vi "ABAPI Dist Exclude Files From Linker Info.vi"(5 "LinkerInfo":T1(array[cluster]), 6 "top-level files":path[](array[path]), 7 "directories of excluded files":string[](array[string])) -> (1 "LinkerInfoOut":T1(array[cluster]), 3 "files excluded":bool)   [LabVIEW 2020]
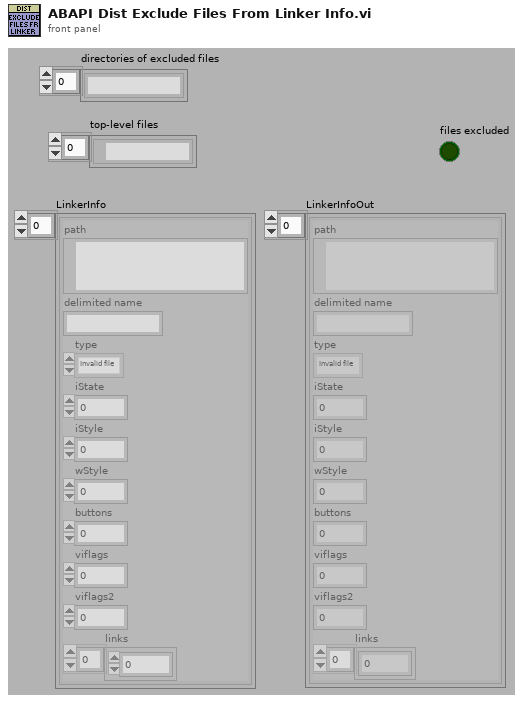
[diagram p1: front panel]
types:
  T1 = cluster{"path":path, "delimited name":string, "type":enum32{"Invalid file", "Unknown type", "Instrument", "Control", "Polymorphic VI", "Project", "Library", "LVClass", "XControl", "XNode", "Shared library", ".NET assembly", "ActiveX interface", "CIN", "Run-time menu", "Palette menu", "Help file", "LLB"}, "iState":u32, "iStyle":u16, "wStyle":u16, "buttons":u16, "viflags":u32, "viflags2":u32, "links":u32[]}[]
  T2 = cluster{"path":path, "delimited name":string, "type":enum32{"Invalid file", "Unknown type", "Instrument", "Control", "Polymorphic VI", "Project", "Library", "LVClass", "XControl", "XNode", "Shared library", ".NET assembly", "ActiveX interface", "CIN", "Run-time menu", "Palette menu", "Help file", "LLB"}, "iState":u32, "iStyle":u16, "wStyle":u16, "buttons":u16, "viflags":u32, "viflags2":u32, "links":u32[]}
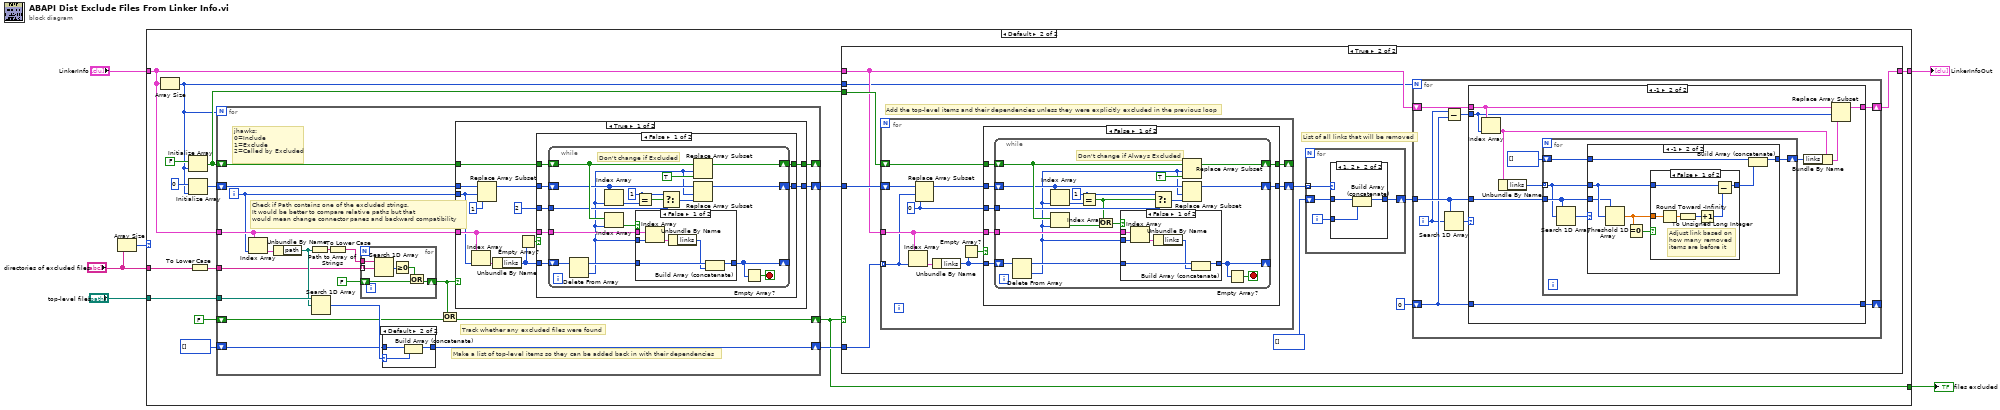
[diagram p0: block diagram]
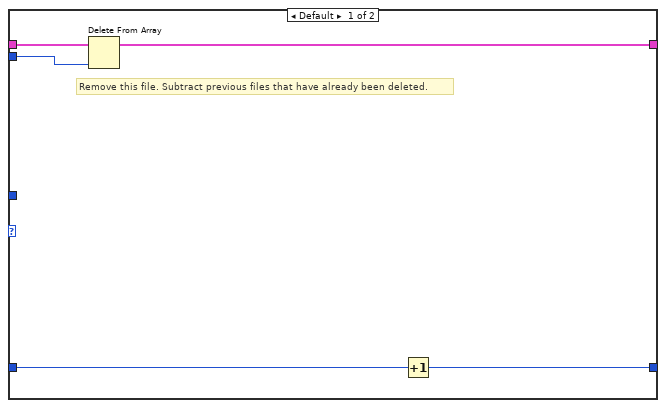
[diagram p4: hidden frame]
diagram:
  n1 = Array Size(array="directories of excluded files") -> (size(s)=w4:i32)
  n2 = case shown="Default" w4 {
    tunnel: "top-level files" -> [_ w19]
    tunnel: [w7 w14] -> w6
    tunnel: "LinkerInfo" -> [w7 w11]
    tunnel: [_ w9] -> w1
    tunnel: "directories of excluded files" -> [_ w8]
    frame 0 {
    }
    frame Default {
      n3 = Array Size(array=w11) -> (size(s)=w13:i32)
      n4 = Initialize Array(FALSE, w13) -> (w16:bool[])
      n5 = Initialize Array(0, w13) -> (w21:i32[])
      n6 = To Lower Case(string=w8) -> (all lower case string=w10:string[])
      n7 = for {
        N: w13 -> [_]
        shift-right: [w138] -> w17
        shift-left: w21 -> [w147]
        shift-right: [w139] -> _
        shift-left: w16 -> [w148]
        tunnel: w11 -> [w146]
        tunnel: w19 -> [w144]
        shift-right: [w142] -> w15
        shift-left: i32[] [] -> [w141]
        shift-right: [w136] -> w9
        shift-left: FALSE -> [w137]
        tunnel: w10 -> [w131]
        i -> [w140]
        # "jhawks:\n0=Include\n1=Exclude\n2=Called by Excluded"
        # "Make a list of top-level items so they can be added back in with their dependencies"
        # "Track whether any excluded files were found"
        # "Check if Path contains one of the excluded strings.\nIt would be better to compare relative paths but that\nwould mean change connector panes and backward compatibility"
        n8 = Index Array(array=w146, index=w140) -> (element=w145:T2)
        n9 = Unbundle By Name(w145) -> ("path"=w132:path)
        n10 = Path to Array of Strings(0:w132) -> (2:w133:string[])  [unwired: 1 out]
        n11 = Search 1D Array(1D array=w144, element=w132) -> (index of element=w143:i32)  [unwired: 1 in]
        n12 = To Lower Case(string=w133) -> (all lower case string=w130:string[])
        n13 = for {
          tunnel: w131 -> [w149] mode=indexing
          tunnel: w130 -> [w152]
          shift-right: [w154] -> w134
          shift-left: FALSE -> [w153]
          n14 = Search 1D Array(1D array=w152, element=w149) -> (index of element=w151:i32)  [unwired: 1 in]
          n15 = Greater Or Equal To 0?(x=w151) -> (x >= 0?=w150:bool)
          n16 = Or(x=w150, y=w153) -> (x .or. y?=w154:bool)
        }
        n17 = case shown="Default" w143 {
          selector: w143 -> [_ w158]
          tunnel: [w155 w157] -> w142
          tunnel: w141 -> [w155 w156]
          frame -1 {
          }
          frame Default {
            n18 = Build Array (concatenate)(w156, w158) -> (w157:i32[])
          }
        }
        n19 = Or(x=w134, y=w137) -> (x .or. y?=w136:bool)
        n20 = case shown="True" w134 {
          tunnel: w146 -> [w165 _]
          tunnel: w147 -> [w169 w205]
          tunnel: [w166 w205] -> w138
          tunnel: w148 -> [w164 w204]
          tunnel: [w163 w204] -> w139
          tunnel: w140 -> [w161 _]
          frame True {
            n21 = Index Array(array=w165, index=w161) -> (element=w170:T2)
            n22 = Replace Array Subset(array=w169, new element=1 ("new element/subarray"), index=w161) -> (w168:i32[])
            n23 = Unbundle By Name(w170) -> ("links"=w160:u32[])
            n24 = Empty Array?(array=w160) -> (empty?=w159:bool)
            n25 = case shown="False" w159 {
              tunnel: w160 -> [w177 _]
              tunnel: w168 -> [w176 w202]
              tunnel: [w175 w202] -> w166
              tunnel: w165 -> [w174 _]
              tunnel: w164 -> [w173 w203]
              tunnel: [w172 w203] -> w163
              tunnel: 2 ("new element/subarray") -> [w171 _]
              frame False {
                n26 = while {
                  shift-right: [w194] -> w175
                  shift-left: w176 -> [w184]
                  tunnel: w171 -> [w180]
                  shift-right: [w190] -> _
                  shift-left: w177 -> [w193]
                  tunnel: w174 -> [w192]
                  shift-right: [w188] -> w172
                  shift-left: w173 -> [w186]
                  stop <- w189 stop-if-true
                  w181 = 1 ("x")
                  # "Don't change if Excluded"
                  n27 = Delete From Array(array=w193) -> (deleted portion=w178:u32, array with subset deleted=w191:u32[])  [unwired: 2 in]
                  n28 = Index Array(array=w184, index=w178) -> (element=w183:i32)
                  n29 = Index Array(array=w186, index=w178) -> (element=w185:bool)
                  n30 = case shown="False" w185 {
                    tunnel: w192 -> [w200 _]
                    tunnel: w178 -> [w199 _]
                    tunnel: w191 -> [w197 w201]
                    tunnel: [w195 w201] -> w190
                    frame False {
                      n31 = Index Array(array=w200, index=w199) -> (element=w198:T2)
                      n32 = Unbundle By Name(w198) -> ("links"=w196:u32[])
                      n33 = Build Array (concatenate)(w197, w196) -> (w195:u32[])
                    }
                    frame True {
                    }
                  }
                  n34 = Equal?(x=w181, y=w183) -> (x = y?=w182:bool)
                  n35 = Select(t=w181, s=w182, f=w180) -> (s? t:f=w179:i32)
                  n36 = Replace Array Subset(array=w186, new element=TRUE ("new element/subarray"), index=w178) -> (w188:bool[])
                  n37 = Replace Array Subset(array=w184, new element=w179, index=w178) -> (w194:i32[])
                  n38 = Empty Array?(array=w190) -> (empty?=w189:bool)
                }
              }
              frame True {
              }
            }
          }
          frame False {
          }
        }
      }
      n39 = case shown="True" w9 {
        tunnel: w17 -> [_ w33]
        tunnel: w16 -> [_ w32]
        tunnel: w15 -> [_ w31]
        tunnel: w11 -> [w23 w27]
        tunnel: [w23 w26] -> w14
        tunnel: w13 -> [_ w25]
        frame False {
        }
        frame True {
          # "List of all links that will be removed"
          # "Add the top-level items and their dependencies unless they were explicitly excluded in the previous loop"
          n40 = for {
            tunnel: w27 -> [w94]
            shift-right: [w95] -> w30
            shift-left: w33 -> [w91]
            shift-right: [w88] -> _
            shift-left: w32 -> [w89]
            tunnel: w31 -> [w87] mode=indexing
            w92 = 0 ("new element/subarray")
            n41 = Index Array(array=w94, index=w87) -> (element=w93:T2)
            n42 = Replace Array Subset(array=w91, new element=w92, index=w87) -> (w90:i32[])
            n43 = Unbundle By Name(w93) -> ("links"=w86:u32[])
            n44 = Empty Array?(array=w86) -> (empty?=w85:bool)
            n45 = case shown="False" w85 {
              tunnel: [w102 w128] -> w95
              tunnel: w94 -> [w101 _]
              tunnel: w86 -> [w100 _]
              tunnel: w92 -> [w99 _]
              tunnel: w90 -> [w98 w128]
              tunnel: w89 -> [w97 w129]
              tunnel: [w96 w129] -> w88
              frame False {
                n46 = while {
                  shift-right: [w118] -> w102
                  shift-left: w98 -> [w109]
                  tunnel: w99 -> [w108]
                  shift-right: [w115] -> _
                  shift-left: w100 -> [w120]
                  tunnel: w101 -> [w117]
                  shift-right: [w114] -> w96
                  shift-left: w97 -> [w112]
                  stop <- w119 stop-if-true
                  w111 = 1 ("x")
                  # "Don't change if Always Excluded"
                  n47 = Delete From Array(array=w120) -> (deleted portion=w106:u32, array with subset deleted=w116:u32[])  [unwired: 2 in]
                  n48 = Index Array(array=w109, index=w106) -> (element=w110:i32)
                  n49 = Index Array(array=w112, index=w106) -> (element=w105:bool)
                  n50 = Equal?(x=w111, y=w110) -> (x = y?=w103:bool)
                  n51 = Or(x=w103, y=w105) -> (x .or. y?=w104:bool)
                  n52 = case shown="False" w104 {
                    tunnel: w117 -> [w126 _]
                    tunnel: w106 -> [w125 _]
                    tunnel: w116 -> [w123 w127]
                    tunnel: [w121 w127] -> w115
                    frame False {
                      n53 = Index Array(array=w126, index=w125) -> (element=w124:T2)
                      n54 = Unbundle By Name(w124) -> ("links"=w122:u32[])
                      n55 = Build Array (concatenate)(w123, w122) -> (w121:u32[])
                    }
                    frame True {
                    }
                  }
                  n56 = Select(t=w111, s=w103, f=w108) -> (s? t:f=w107:i32)
                  n57 = Replace Array Subset(array=w112, new element=TRUE ("new element/subarray"), index=w106) -> (w114:bool[])
                  n58 = Replace Array Subset(array=w109, new element=w107, index=w106) -> (w118:i32[])
                  n59 = Empty Array?(array=w115) -> (empty?=w119:bool)
                }
              }
              frame True {
              }
            }
          }
          n60 = for {
            tunnel: w30 -> [w80] mode=indexing
            shift-right: [w78] -> w28
            shift-left: i32[] [] -> [w77]
            i -> [w79]
            n61 = case shown="1, 2" w80 {
              tunnel: w79 -> [_ w84]
              tunnel: [w81 w83] -> w78
              tunnel: w77 -> [w81 w82]
              frame 0, Default {
              }
              frame 1, 2 {
                n62 = Build Array (concatenate)(w82, w84) -> (w83:i32[])
              }
            }
          }
          n63 = for {
            N: w25 -> [_]
            tunnel: w28 -> [w41]
            shift-right: [w38] -> w26
            shift-left: w27 -> [w39]
            shift-right: [w37] -> _
            shift-left: 0 -> [w36]
            i -> [w35]
            n64 = Subtract(x=w35, y=w36) -> (x-y=w34:i32)
            n65 = Search 1D Array(1D array=w41, element=w35) -> (index of element=w40:i32)  [unwired: 1 in]
            n66 = case shown="-1" w40 {
              tunnel: w41 -> [_ w56]
              tunnel: w39 -> [w46 w51]
              tunnel: [w45 w49] -> w38
              tunnel: w34 -> [w42 w47]
              tunnel: [w44 w48] -> w37
              tunnel: w36 -> [w43 w48]
              frame Default {
                # "Remove this file. Subtract previous files that have already been deleted."
                n67 = Delete From Array(array=w46, index=w42) -> (array with subset deleted=w45:T1)  [unwired: 1 in, 1 out]
                n68 = Increment(x=w43) -> (x+1=w44:i32)
              }
              frame -1 {
                n69 = Index Array(array=w51, index=w47) -> (element=w53:T2)
                n70 = Unbundle By Name(w53) -> ("links"=w54:u32[])
                n71 = for {
                  tunnel: w54 -> [w57] mode=indexing
                  shift-right: [w59] -> w52
                  shift-left: u32[] [] -> [w58]
                  tunnel: w56 -> [w61]
                  n72 = Search 1D Array(1D array=w61, element=w57) -> (index of element=w60:i32)  [unwired: 1 in]
                  n73 = case shown="-1" w60 {
                    tunnel: w57 -> [_ w67]
                    tunnel: w61 -> [_ w66]
                    tunnel: [w62 w64] -> w59
                    tunnel: w58 -> [w62 w63]
                    frame Default {
                      # "This index points to a file being removed."
                    }
                    frame -1 {
                      n74 = Threshold 1D Array(2:w67, 3:w66) -> (0:w69:dbl)  [unwired: 1 in]
                      n75 = Equal To 0?(x=w69) -> (x = 0?=w68:bool)
                      n76 = case shown="False" w68 {
                        tunnel: [w72 w76] -> w65
                        tunnel: w69 -> [w74 _]
                        tunnel: w67 -> [w73 w76]
                        frame False {
                          # "Adjust link based on\nhow many removed\nitems are before it"
                          n77 = Round Toward -Infinity(1:w74) -> (0:w75:dbl)
                          n78 = To Unsigned Long Integer(number=w75) -> (unsigned 32bit integer=w71:u32)
                          n79 = Increment(x=w71) -> (x+1=w70:u32)
                          n80 = Subtract(x=w73, y=w70) -> (x-y=w72:u32)
                        }
                        frame True {
                          # "This link is before \nany deleted items"
                        }
                      }
                      n81 = Build Array (concatenate)(w63, w65) -> (w64:u32[])
                    }
                  }
                }
                n82 = Bundle By Name(cluster=w53, "links"=w52) -> (w50:T2)
                n83 = Replace Array Subset(array=w51, new element=w50, index=w47) -> (w49:T1)
              }
            }
          }
        }
      }
    }
  }
  "LinkerInfoOut" <- w6
  "files excluded" <- w1
